vi "34970 Read Scanned Data v2.vi"(3 "error out":errorcluster, 4 "# Channels":u32, 5 "VISA session 2":refnum<visa-resource-name>) -> (0 "error":errorcluster, 1 "Data String":string, 2 "VISA Resource Name":refnum<visa-resource-name>)   [LabVIEW 2020]
doc: "Used with preconfigured scans and 34970 Query # Channel Readings. Fetches completed scan data when query says they are ready. Saves CPU time compared to MEASure commands by not issuing VISA read until all readings are ready in 34970 onboard memory.\nW. Gilbert, University of Minnesota Physics, 8/6/2004\nwgilbert@physics.umn.edu"
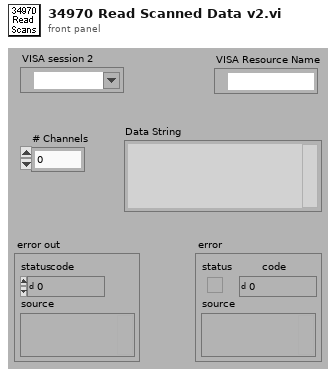
[diagram p1: front panel]
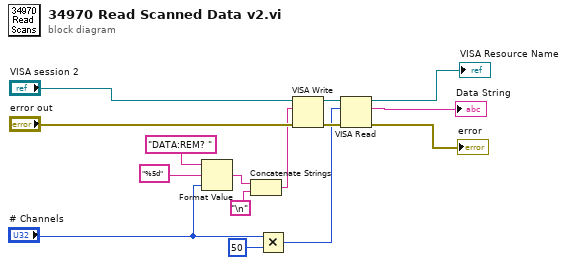
[diagram p0: block diagram]
diagram:
  n1 = Format Value(string ("")="DATA:REM? ", format string="%5d", value (0)="# Channels") -> (output string=w9:string)
  n2 = Concatenate Strings(w9, "\n") -> (w10:string)
  n3 = Multiply(x="# Channels", y=u32 50) -> (x*y=w1:u32)
  n4 = VISA Write(VISA resource name="VISA session 2", write buffer=w10, error in (no error)="error out") -> (VISA resource name out=w5:refnum<visa-resource-name>, error out=w6:errorcluster)  [unwired: 1 out]
  n5 = VISA Read(VISA resource name=w5, byte count=w1, error in (no error)=w6) -> (VISA resource name out=→"VISA Resource Name":refnum<visa-resource-name>, read buffer=→"Data String":string, error out=→"error":errorcluster)  [unwired: 1 out]
